vi "_Lookup Double Group.vi"(8 "error in (no error)":errorcluster, 10 "Group Name":string, 11 "Loop Data in":T1) -> (0 "error out":errorcluster, 2 "Group":refnum<class "GroupAbstract.lvclass">, 3 "Loop Data":T1)   [LabVIEW 2020, in "Vecto.lvlib" / "ChannelService.lvclass"]
uses:
  ChannelService.lvclass
  Loop Data.ctl
  GroupAbstract/GroupAbstract.lvclass
  ChannelService.lvclass/ChannelService.ctl
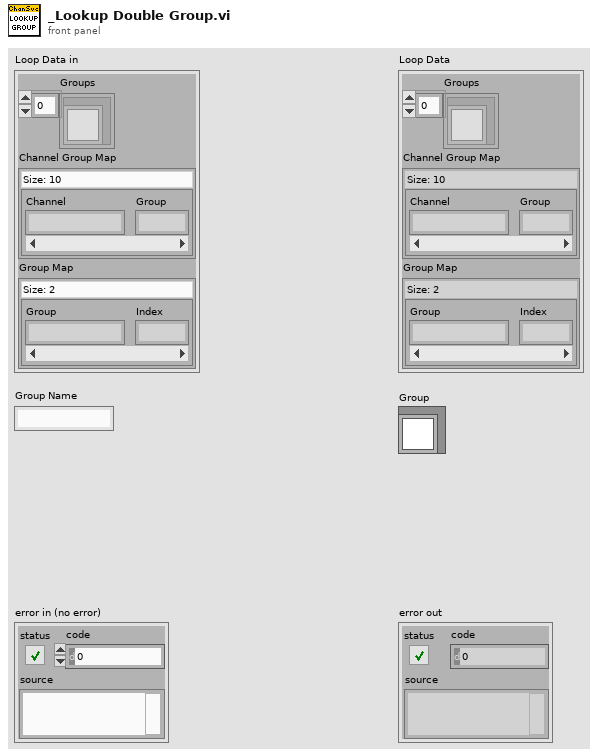
[diagram p1: front panel]
types:
  T1 = typedef "Vecto.lvlib/ChannelService.lvclass/Loop Data.ctl" = cluster{"Groups":refnum<class "GroupAbstract.lvclass">[], "Channel Group Map":map{string, i32}, "Group Map":map{string, i32}}
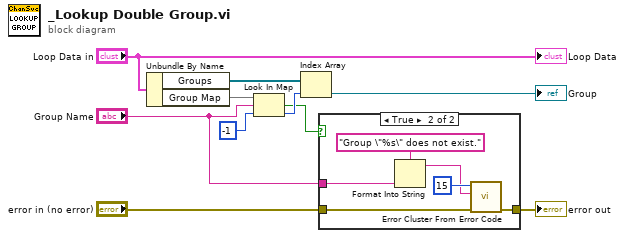
[diagram p0: block diagram]
diagram:
  n1 = Unbundle By Name("Loop Data in") -> ("Groups"=w8:refnum<class "GroupAbstract.lvclass">[], "Group Map"=w9:map{string, i32})
  n2 = Look In Map(map=w9, key="Group Name", default value=-1) -> (key not found?=w5:bool, value=w6:i32)
  n3 = Index Array(array=w8, index=w6) -> (element=→"Group":refnum<class "GroupAbstract.lvclass">)
  n4 = case shown="True" w5 {
    tunnel: "error in (no error)" -> [w11 w17]
    tunnel: [w11 w16] -> w1
    tunnel: "Group Name" -> [_ w12]
    frame False {
    }
    frame True {
      n5 = Format Into String(format string="Group \"%s\" does not exist.", w12) -> (resulting string=w13:string)  [unwired: 2 in, 1 out]
      n6 = call <vilib>:"Error Cluster From Error Code.vi"("error in (no error)"=w17, "error message (\"\")"=w13, "error code (0)"=15) -> ("error out"=w16:errorcluster)  [unwired: 6 in]
    }
  }
  "error out" <- w1
  "Loop Data" <- "Loop Data in"
